vi "Accuracy.vi"(10 "Y":sgl[](array[numeric]), 11 "Yref":sgl) -> (3 "Accuracy":sgl)   [LabVIEW 2020, in "EPA 1065.lvlib" / "ARN Test 1065-305.lvlib"]
uses:
  ARN Test 1065-305.lvlib
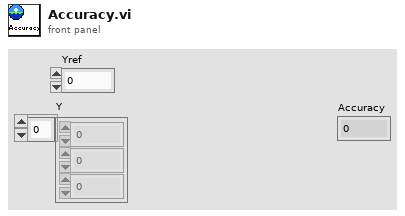
[diagram p1: front panel]
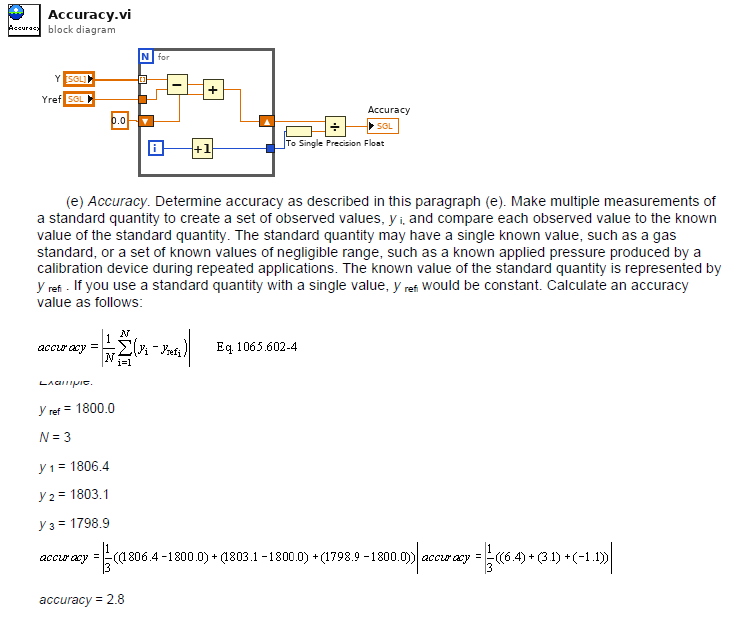
[diagram p0: block diagram]
diagram:
  n1 = for {
    tunnel: "Y" -> [w11] mode=indexing
    tunnel: [w13] -> w3
    tunnel: "Yref" -> [w12]
    shift-right: [w9] -> w4
    shift-left: sgl 0.0 -> [w8]
    i -> [w14]
    n2 = Subtract(x=w11, y=w12) -> (x-y=w10:sgl)
    n3 = Increment(x=w14) -> (x+1=w13:i32)
    n4 = Add(x=w10, y=w8) -> (x+y=w9:sgl)
  }
  n5 = To Single Precision Float(number=w3) -> (single precision float=w2:sgl)
  n6 = Divide(x=w4, y=w2) -> (x/y=→"Accuracy":sgl)
